vi "XY Graph Fold Plot xn.vi"(8 "Error In":errorcluster, 9 "Message in":string, 10 "# Folds":u32=1 min=1, 11 "Decay (in) in":cluster{"X Axis":dbl[], "Y Axis":dbl[]}) -> (0 "Error Out":errorcluster, 1 "Message out":string, 2 "# Folds (actual)":u32=1 min=1, 3 "Decay (in) out":cluster{"X Axis":dbl[], "Y Axis":dbl[]})   [LabVIEW 2021, in "XY Graph Add-Ons.lvlib"]
uses:
  XY Graph Add-Ons.lvlib
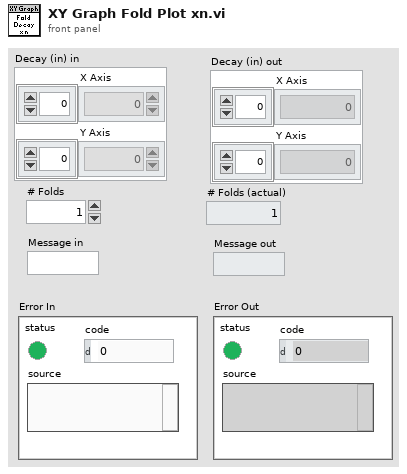
[diagram p1: front panel]
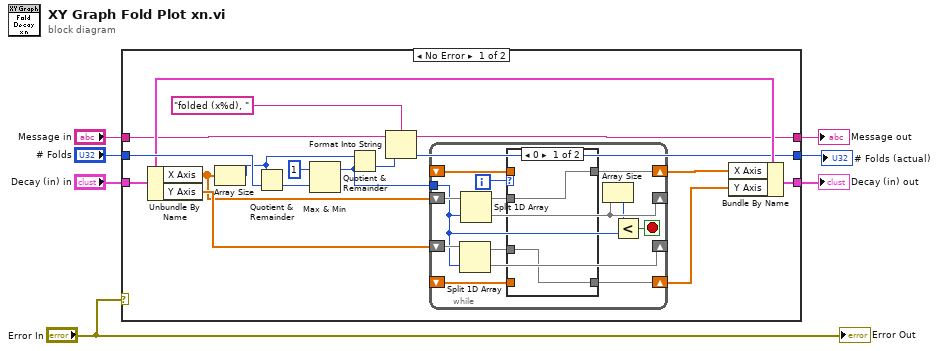
[diagram p0: block diagram]
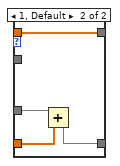
[diagram p2: hidden frame]
diagram:
  n1 = case shown="No Error" "Error In" {
    tunnel: "# Folds" -> [w22 w43]
    tunnel: [w21 w44] -> w6
    tunnel: "Decay (in) in" -> [w18 w44]
    tunnel: [w14 w45] -> w4
    tunnel: "Message in" -> [w12 w45]
    tunnel: [w9 w43] -> w1
    frame No Error {
      n2 = Unbundle By Name(w18) -> ("X Axis"=w15:dbl[], "Y Axis"=w16:dbl[])
      n3 = Array Size(array=w15) -> (size(s)=w8:i32)
      n4 = Quotient & Remainder(x=w8, y=w22) -> (floor(x/y)=w17:u32)  [unwired: 1 out]
      n5 = Max & Min(x=u32 1, y=w17) -> (max(x,y)=w10:u32)  [unwired: 1 out]
      n6 = Quotient & Remainder(x=w8, y=w10) -> (floor(x/y)=w9:u32)  [unwired: 1 out]
      n7 = Format Into String(format string="folded (x%d), ", initial string=w12, w9) -> (resulting string=w14:string)  [unwired: 1 in, 1 out]
      n8 = while {
        shift-right: [w26] -> _
        shift-left: w15 -> [w36]
        shift-right: [w27] -> _
        shift-left: w16 -> [w35]
        tunnel: w10 -> [w23]
        shift-right: [w33] -> w20
        shift-left: _ -> [w31]
        shift-right: [w29] -> w19
        shift-left: _ -> [w28]
        i -> [w34]
        stop <- w24 stop-if-true
        n9 = Split 1D Array(array=w35, index=w23) -> (first subarray=w32:dbl[], second subarray=w27:dbl[])
        n10 = Split 1D Array(array=w36, index=w23) -> (first subarray=w30:dbl[], second subarray=w26:dbl[])
        n11 = case shown="0" w34 {
          tunnel: [w38 w40] -> w33
          tunnel: w32 -> [w38 w42]
          tunnel: w31 -> [_ w41]
          tunnel: w30 -> [w37 _]
          tunnel: [w37 w39] -> w29
          tunnel: w28 -> [_ w39]
          frame 0 {
          }
          frame 1, Default {
            n12 = Add(x=w42, y=w41) -> (x+y=w40:dbl[])
          }
        }
        n13 = Array Size(array=w26) -> (size(s)=w25:i32)
        n14 = Less?(x=w25, y=w23) -> (x < y?=w24:bool)
      }
      n15 = Bundle By Name(cluster=w18, "X Axis"=w19, "Y Axis"=w20) -> (w21:cluster{"X Axis":dbl[], "Y Axis":dbl[]})
    }
    frame Error {
    }
  }
  "Decay (in) out" <- w6
  "Message out" <- w4
  "# Folds (actual)" <- w1
  "Error Out" <- "Error In"
